vi "CollectData.vi"(8 "error in (no error)":errorcluster, 11 "Pulseblaster in":refnum<class "Pulseblaster.lvclass">) -> (0 "error out":errorcluster, 3 "Pulseblaster out":refnum<class "Pulseblaster.lvclass">)   [LabVIEW 2013, in "Pulseblaster.lvclass"]
uses:
  Pulseblaster.lvclass
  Master Device/Master Device.lvclass
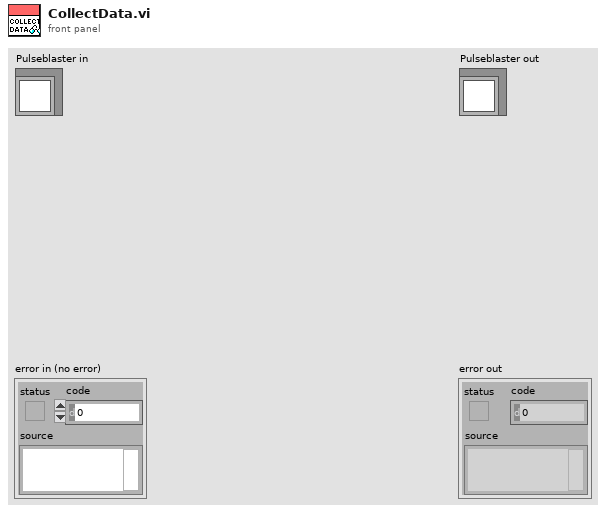
[diagram p1: front panel]
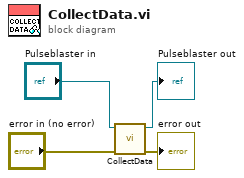
[diagram p0: block diagram]
diagram:
  n1 = call-parent "CollectData.vi"("error in (no error)"="error in (no error)", "Master Device in"="Pulseblaster in") -> ("error out"=→"error out":errorcluster, "Master Device out"=→"Pulseblaster out":refnum<class "Pulseblaster.lvclass">)  [unwired: 8 in]
